vi "SGLToU32.vi"(11 "SGL":sgl format="%#.6f") -> (3 "U32":u32)   [LabVIEW 2016]
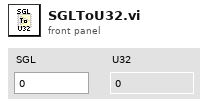
[diagram p1: front panel]
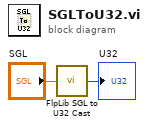
[diagram p0: block diagram]
diagram:
  n1 = call <userlib>:"FlpLib SGL to U32 Cast.vi"("x"="SGL") -> ("y"=→"U32":u32)  [unwired: 4 in]
